vi "Try Add.vi"(8 "error in":errorcluster, 9 "Sub Object":refnum<class "Sub Object.lvclass">, 10 "Sub Index":u8, 11 "Sub Objects Dictionary in":refnum<class "Sub Objects Dictionary.lvclass">) -> (0 "error out":errorcluster, 2 "Success":bool, 3 "Sub Objects Dictionary out":refnum<class "Sub Objects Dictionary.lvclass">)   [LabVIEW 2020, in "CANopen.lvlib" / "Sub Objects Dictionary.lvclass"]
doc: "Attempts to add the specified key and value to the dictionary."
uses:
  Sub Objects Dictionary.lvclass
  Sub Objects Dictionary.lvclass/Sub Objects Dictionary.ctl
  Sub Object/Sub Object.lvclass
  Ordered-Dictionary/Ordered Object Dictionary/Source/Ordered Object Dictionary.lvclass
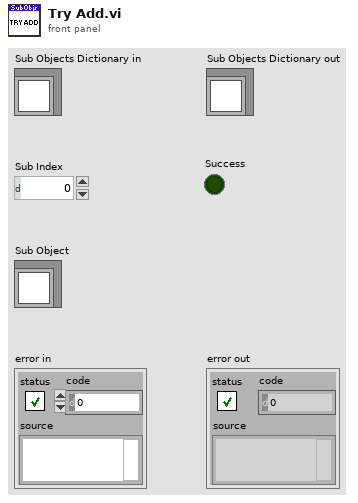
[diagram p1: front panel]
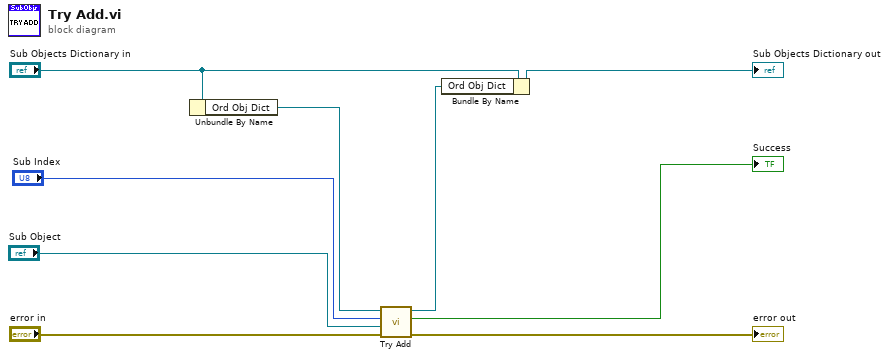
[diagram p0: block diagram]
diagram:
  n1 = Unbundle By Name("Sub Objects Dictionary in") -> ("Ord Obj Dict"=w6:refnum<class "Ordered Object Dictionary.lvclass">)
  n2 = call "Try Add.vi"("error in"="error in", "Value"="Sub Object", "Key"="Sub Index", "Ordered Object Dictionary in"=w6) -> ("error out"=→"error out":errorcluster, "Success"=→"Success":bool, "Ordered Object Dictionary out"=w2:refnum<class "Ordered Object Dictionary.lvclass">)  [unwired: 5 in]
  n3 = Bundle By Name(cluster="Sub Objects Dictionary in", "Ord Obj Dict"=w2) -> (→"Sub Objects Dictionary out":refnum<class "Sub Objects Dictionary.lvclass">)
